vi "Example - GUI.vi"() -> ()   [LabVIEW 2016, in "Global_logger.lvlib"]
doc: "Example of logging into UI elements."
uses:
  Global_logger.lvlib
  UI Options.ctl
  New UI Logger.vi
panel:
  in  "Table Control":string[][](table)
  in  "Multicolumn Listbox":i32(listbox)=-1
  in  "Listbox":i32(listbox)=-1
  in  "String":string
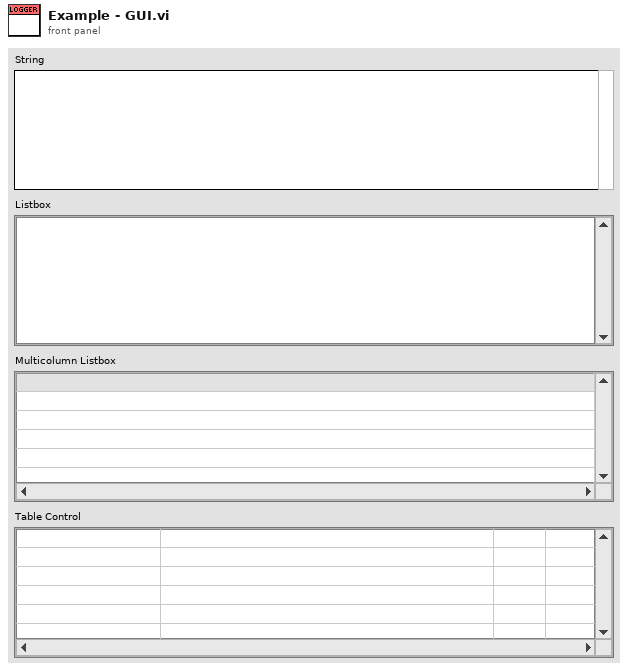
[diagram p1: front panel]
types:
  T1 = typedef "Global_logger.lvlib/UI Options.ctl" = cluster{"Ctl Refnum":refnum<vi>, "Delimiter":string}
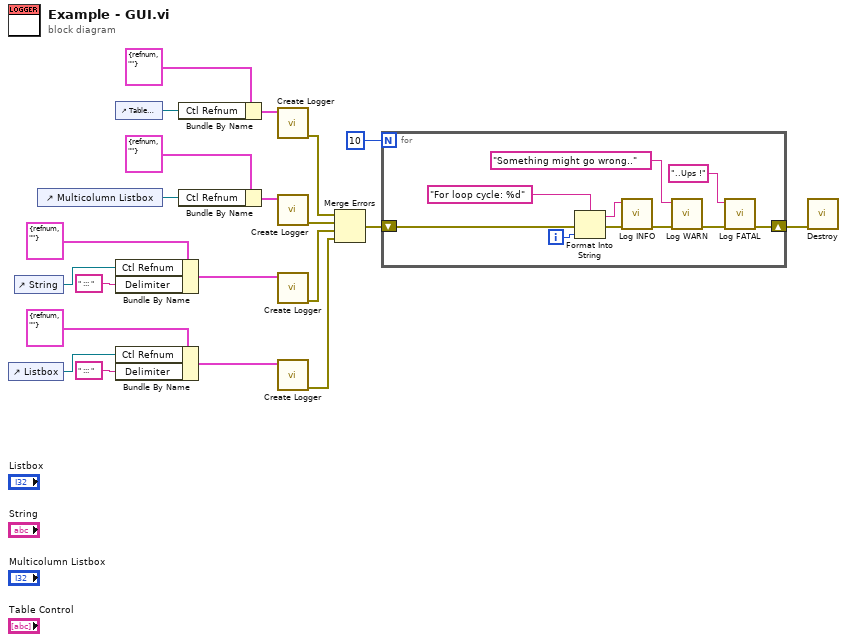
[diagram p0: block diagram]
diagram:
  n1 = control-ref of="Listbox"() -> (w15:refnum<vi>)
  n2 = control-ref of="String"() -> (w18:refnum<vi>)
  n3 = control-ref of="Multicolumn Listbox"() -> (w14:refnum<vi>)
  n4 = control-ref of="Table Control"() -> (w11:refnum<vi>)
  n5 = Bundle By Name(cluster=T1 {"Ctl Refnum"=refnum, "Delimiter"=""} ("UI Options"), "Ctl Refnum"=w18, "Delimiter"=" ::: ") -> (w19:T1)
  n6 = Bundle By Name(cluster=T1 {"Ctl Refnum"=refnum, "Delimiter"=""} ("UI Options"), "Ctl Refnum"=w15, "Delimiter"=" ::: ") -> (w16:T1)
  n7 = Bundle By Name(cluster=T1 {"Ctl Refnum"=refnum, "Delimiter"=""} ("UI Options"), "Ctl Refnum"=w11) -> (w10:T1)
  n8 = Bundle By Name(cluster=T1 {"Ctl Refnum"=refnum, "Delimiter"=""} ("UI Options"), "Ctl Refnum"=w14) -> (w13:T1)
  n9 = call-poly "Create Logger.vi"("UI Options"=w10) -> ("error out"=w5:errorcluster)  [unwired: 10 in]
  n10 = call-poly "Create Logger.vi"("UI Options"=w13) -> ("error out"=w4:errorcluster)  [unwired: 10 in]
  n11 = call-poly "Create Logger.vi"("UI Options"=w19) -> ("error out"=w3:errorcluster)  [unwired: 10 in]
  n12 = call-poly "Create Logger.vi"("UI Options"=w16) -> ("error out"=w2:errorcluster)  [unwired: 10 in]
  n13 = Merge Errors(w5, w4, w3, w2) -> (w1:errorcluster)
  n14 = for {
    N: 10 -> [_]
    shift-right: [w30] -> w21
    shift-left: w1 -> [w22]
    i -> [w27]
    n15 = Format Into String(format string="For loop cycle: %d", error in=w22, w27) -> (resulting string=w25:string, error out=w28:errorcluster)  [unwired: 1 in]
    n16 = call "Log INFO.vi"("error in (no error)"=w28, "Message"=w25) -> ("error out"=w31:errorcluster)  [unwired: 9 in]
    n17 = call "Log WARN.vi"("error in (no error)"=w31, "Message"="Something might go wrong.." ("format string")) -> ("error out"=w24:errorcluster)  [unwired: 9 in]
    n18 = call "Log FATAL.vi"("error in (no error)"=w24, "Message"="..Ups !") -> ("error out"=w30:errorcluster)  [unwired: 9 in]
  }
  n19 = call "Destroy.vi"("error in (no error)"=w21) -> ()  [unwired: 10 in, 1 out]
